vi "打开仪器_仪器选择界面.vi"() -> ()   [LabVIEW 2014]
panel:
  in  "仪器选择":enum32{"未选择", "示波器", "多道分析器", "单道分析器", "TDC"}(radio)=enum."示波器"
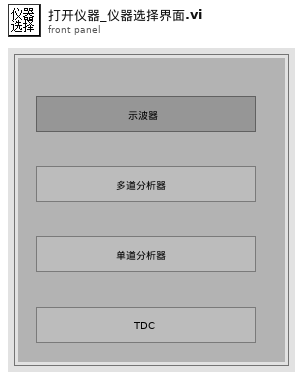
[diagram p1: front panel]
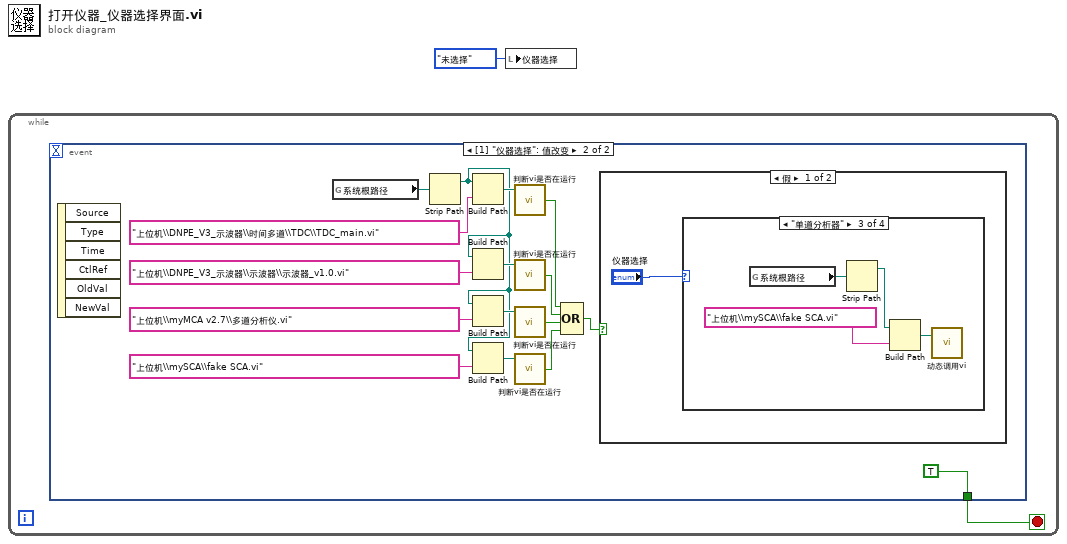
[diagram p0: block diagram]
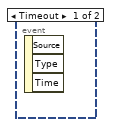
[diagram p2: hidden frame]
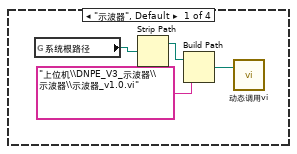
[diagram p3: hidden frame]
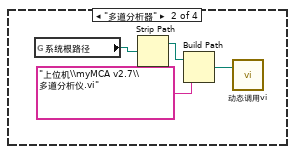
[diagram p4: hidden frame]
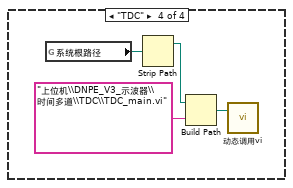
[diagram p5: hidden frame]
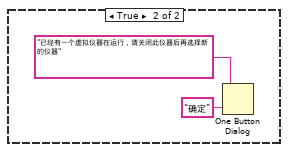
[diagram p6: hidden frame]
diagram:
  n1 = while {
    stop <- w2 stop-if-true
    n2 = event shown="[1] \"仪器选择\": 值改变" {
      selector: _ -> [_ _]
      dyn-events: _ -> [_ _]
      timeout: _ -> [_ _]
      tunnel: [_ TRUE] -> w2
      event Timeout {
        n3 = event-data() -> ()  [unwired: 1 in, 3 out]
      }
      event "仪器选择": Value Change {
        n4 = event-data() -> ()  [unwired: 1 in, 6 out]
        n5 = global read "系统全局变量.vi" "系统根路径"() -> (w18:path)
        n6 = Strip Path(path=w18) -> (stripped path=w4:path)  [unwired: 1 out]
        n7 = Build Path(base path=w4, name or relative path="上位机\\DNPE_V3_示波器\\时间多道\\TDC\\TDC_main.vi" ("名称或相对路径")) -> (appended path=w16:path)
        n8 = Build Path(base path=w4, name or relative path="上位机\\DNPE_V3_示波器\\示波器\\示波器_v1.0.vi" ("名称或相对路径")) -> (appended path=w15:path)
        n9 = Build Path(base path=w4, name or relative path="上位机\\myMCA v2.7\\多道分析仪.vi" ("名称或相对路径")) -> (appended path=w12:path)
        n10 = Build Path(base path=w4, name or relative path="上位机\\mySCA\\fake SCA.vi" ("名称或相对路径")) -> (appended path=w11:path)
        n11 = call "判断vi是否在运行.vi"("VI路径"=w16) -> ("vi正在运行?"=w9:bool)  [unwired: 2 in, 2 out]
        n12 = call "判断vi是否在运行.vi"("VI路径"=w15) -> ("vi正在运行?"=w8:bool)  [unwired: 2 in, 2 out]
        n13 = call "判断vi是否在运行.vi"("VI路径"=w12) -> ("vi正在运行?"=w7:bool)  [unwired: 2 in, 2 out]
        n14 = call "判断vi是否在运行.vi"("VI路径"=w11) -> ("vi正在运行?"=w6:bool)  [unwired: 2 in, 2 out]
        n15 = Compound Arithmetic op=OR(w9, w8, w7, w6) -> (w5:bool)
        n16 = case shown="假" w5 {
          frame False {
            n17 = case shown="\"单道分析器\"" "仪器选择" {
              frame "示波器", Default {
                n18 = global read "系统全局变量.vi" "系统根路径"() -> (w23:path)
                n19 = Strip Path(path=w23) -> (stripped path=w22:path)  [unwired: 1 out]
                n20 = Build Path(base path=w22, name or relative path="上位机\\DNPE_V3_示波器\\示波器\\示波器_v1.0.vi" ("名称或相对路径")) -> (appended path=w20:path)
                n21 = call "动态调用vi.vi"("VI路径"=w20) -> ()  [unwired: 1 in, 1 out]
              }
              frame "多道分析器" {
                n22 = global read "系统全局变量.vi" "系统根路径"() -> (w27:path)
                n23 = Strip Path(path=w27) -> (stripped path=w26:path)  [unwired: 1 out]
                n24 = Build Path(base path=w26, name or relative path="上位机\\myMCA v2.7\\多道分析仪.vi" ("名称或相对路径")) -> (appended path=w24:path)
                n25 = call "动态调用vi.vi"("VI路径"=w24) -> ()  [unwired: 1 in, 1 out]
              }
              frame "单道分析器" {
                n26 = global read "系统全局变量.vi" "系统根路径"() -> (w31:path)
                n27 = Strip Path(path=w31) -> (stripped path=w30:path)  [unwired: 1 out]
                n28 = Build Path(base path=w30, name or relative path="上位机\\mySCA\\fake SCA.vi" ("名称或相对路径")) -> (appended path=w28:path)
                n29 = call "动态调用vi.vi"("VI路径"=w28) -> ()  [unwired: 1 in, 1 out]
              }
              frame "TDC" {
                n30 = global read "系统全局变量.vi" "系统根路径"() -> (w35:path)
                n31 = Strip Path(path=w35) -> (stripped path=w34:path)  [unwired: 1 out]
                n32 = Build Path(base path=w34, name or relative path="上位机\\DNPE_V3_示波器\\时间多道\\TDC\\TDC_main.vi" ("名称或相对路径")) -> (appended path=w32:path)
                n33 = call "动态调用vi.vi"("VI路径"=w32) -> ()  [unwired: 1 in, 1 out]
              }
            }
          }
          frame True {
            n34 = One Button Dialog(message="已经有一个虚拟仪器在运行，请关闭此仪器后再选择新的仪器" ("消息"), button name ("OK")="确定" ("按钮名称（“确定”）")) -> ()  [unwired: 1 out]
          }
        }
      }
    }
  }
  n35 = local write "仪器选择"(enum32{"未选择", "示波器", "多道分析器", "单道分析器", "TDC"}."未选择" ("仪器选择")) -> ()
